vi "Post-Build Action.vi"(5 "Files Generated by Build":path[](array[path]), 6 "Top Level/Always Included VIs":path[](array[path]), 7 "Destination Path":path, 8 "error in (no error)":errorcluster, 9 "Target Name":string, 10 "Build Specification Name":string, 11 "Project Path":path) -> (0 "error out":errorcluster)   [LabVIEW 2015]
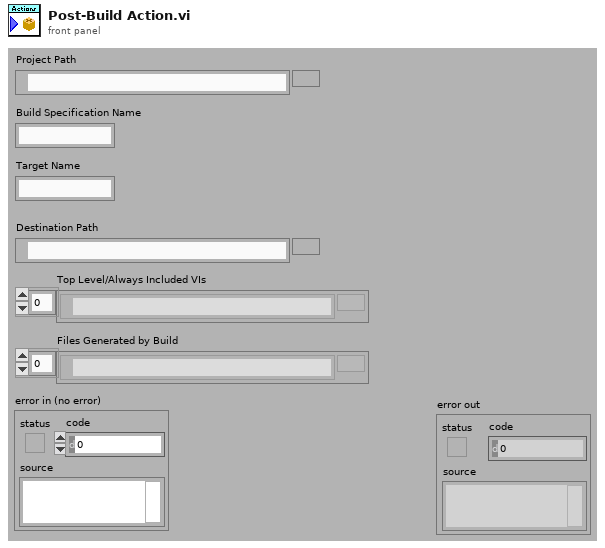
[diagram p1: front panel]
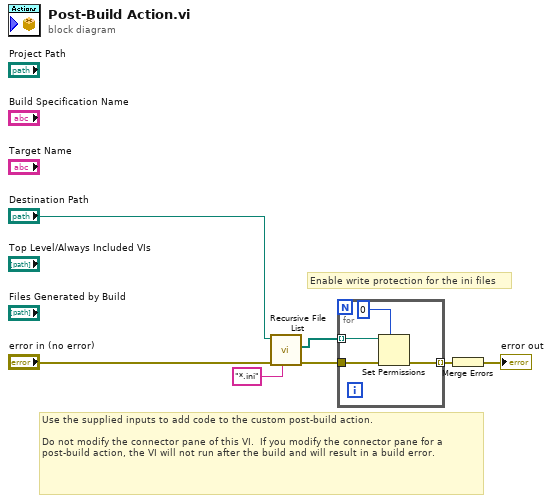
[diagram p0: block diagram]
diagram:
  # "Enable write protection for the ini files"
  # "Use the supplied inputs to add code to the custom post-build action.\n\nDo not modify the connector pane of this VI.  If you modify the connector pane for a post-build action, the VI will not run after the build and will result in a build error."
  n1 = call <vilib>:"Recursive File List.vi"("pattern"="*.ini", "error in (no error)"="error in (no error)", "Folder Path"="Destination Path") -> ("error out"=w4:errorcluster, "All Files in Dir"=w3:path[])  [unwired: 4 in, 3 out]
  n2 = for {
    tunnel: w4 -> [w11]
    tunnel: [w10] -> w2 mode=indexing
    tunnel: w3 -> [w9] mode=indexing
    n3 = Set Permissions(7:i16 0 ("permissions"), 8:w11, 11:w9) -> (0:w10:errorcluster)  [unwired: 2 in, 1 out]
  }
  n4 = Merge Errors(w2) -> (→"error out":errorcluster)
